vi "Init Buffer.vi"(8 "error in (no error)":errorcluster, 11 "ONNX Class in":refnum<class "ONNX Class.lvclass">) -> (0 "error out":errorcluster, 3 "ONNX Class out":refnum<class "ONNX Class.lvclass">)   [LabVIEW 2017, in "ONNX Class Library.lvlib" / "ONNX Class.lvclass"]
uses:
  ONNX Class.lvclass
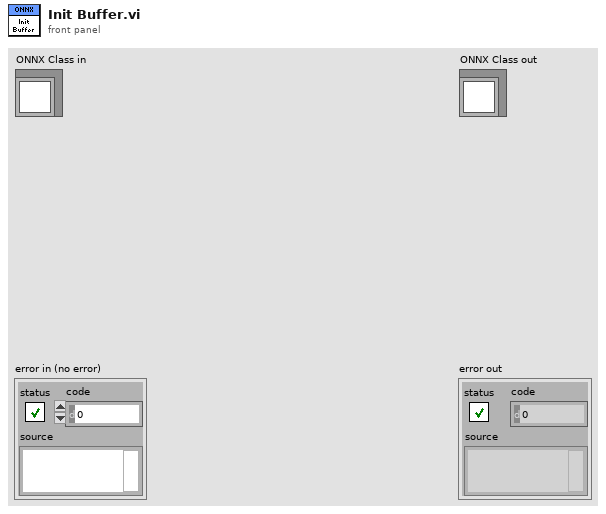
[diagram p1: front panel]
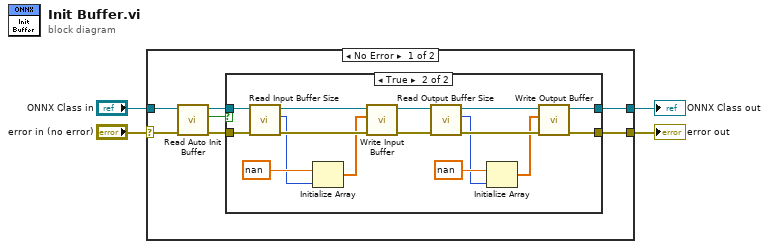
[diagram p0: block diagram]
diagram:
  n1 = case shown="No Error" "error in (no error)" {
    selector: "error in (no error)" -> [w10 w31]
    tunnel: [w5 w31] -> w3
    tunnel: [w6 w30] -> w1
    tunnel: "ONNX Class in" -> [w11 w30]
    frame No Error {
      n2 = call-dynamic "Read Auto Init Buffer.vi"("error in (no error)"=w10, "ONNX Class in"=w11) -> ("error out"=w7:errorcluster, "Auto Init Buffer"=w9:bool, "ONNX Class out"=w8:refnum<class "ONNX Class.lvclass">)  [unwired: 7 in]
      n3 = case shown="True" w9 {
        tunnel: w8 -> [w13 w29]
        tunnel: w7 -> [w12 w28]
        tunnel: [w13 w21] -> w6
        tunnel: [w12 w20] -> w5
        frame False {
        }
        frame True {
          n4 = call-dynamic "Read Input Buffer Size.vi"("error in (no error)"=w28, "ONNX Class in"=w29) -> ("error out"=w26:errorcluster, "Input Buffer Size"=w18:i64, "ONNX Class out"=w27:refnum<class "ONNX Class.lvclass">)  [unwired: 7 in]
          n5 = Initialize Array(sgl nan ("element"), w18) -> (w17:sgl[])
          n6 = call-dynamic "Write Input Buffer.vi"("error in (no error)"=w26, "Input Buffer"=w17, "ONNX Class in"=w27) -> ("error out"=w24:errorcluster, "ONNX Class out"=w25:refnum<class "ONNX Class.lvclass">)  [unwired: 7 in]
          n7 = call-dynamic "Read Output Buffer Size.vi"("error in (no error)"=w24, "ONNX Class in"=w25) -> ("error out"=w22:errorcluster, "Output Buffer Size"=w15:i64, "ONNX Class out"=w23:refnum<class "ONNX Class.lvclass">)  [unwired: 7 in]
          n8 = Initialize Array(sgl nan ("element"), w15) -> (w14:sgl[])
          n9 = call-dynamic "Write Output Buffer.vi"("error in (no error)"=w22, "Output Buffer"=w14, "ONNX Class in"=w23) -> ("error out"=w20:errorcluster, "ONNX Class out"=w21:refnum<class "ONNX Class.lvclass">)  [unwired: 7 in]
        }
      }
    }
    frame Error {
    }
  }
  "error out" <- w3
  "ONNX Class out" <- w1
